vi "Create Virtual Folder (Project Item In).vi"(8 "error in":errorcluster, 10 "Item to Find":string, 11 "ProjectItem In":refnum<vi>) -> (0 "error out":errorcluster, 3 "ProjectItem out":refnum<vi>)   [LabVIEW 2014, in "SPI Engine Scripting.lvlib"]
uses:
  SPI Engine Scripting.lvlib
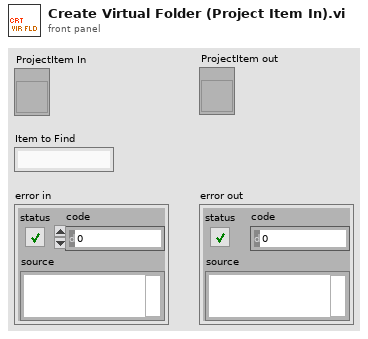
[diagram p1: front panel]
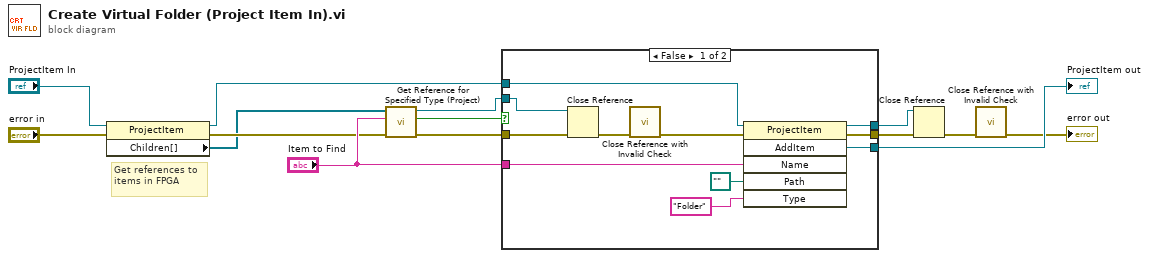
[diagram p0: block diagram]
diagram:
  # "Get references to items in FPGA"
  n1 = property class="ProjectItem"(reference="ProjectItem In", error in="error in") -> (reference out=w3:refnum<vi>, error out=w11:errorcluster, "Children[]"=w7:refnum<vi>[])
  n2 = call "Get Reference for Specified Type (Project).vi"("error in (no error)"=w11, "Type to Find"="Item to Find", "Array of References"=w7) -> ("error out"=w9:errorcluster, "Item Found"=w8:bool, "Project Item"=w10:refnum<vi>)  [unwired: 6 in]
  n3 = case shown="False" w8 {
    tunnel: [w21 w27] -> w14
    tunnel: w9 -> [w17 w28]
    tunnel: w10 -> [w15 w27]
    tunnel: [w22 w28] -> w5
    tunnel: "Item to Find" -> [w23 _]
    tunnel: [w20 w26] -> w4
    tunnel: w3 -> [w19 w26]
    frame False {
      n4 = Close Reference(reference=w15, error in (no error)=w17) -> (error out=w18:errorcluster)
      n5 = call "Close Reference with Invalid Check.vi"("error in (no error)"=w18) -> ("error out"=w16:errorcluster)  [unwired: 10 in]
      n6 = invoke class="ProjectItem" method="AddItem"(reference=w19, error in=w16, "Name"=w23, "Path"=path "", "Type"="Folder") -> (reference out=w20:refnum<vi>, error out=w22:errorcluster, "AddItem"=w21:refnum<vi>)  [unwired: 1 in, 3 out]
    }
    frame True {
    }
  }
  "ProjectItem out" <- w14
  n7 = Close Reference(reference=w4, error in (no error)=w5) -> (error out=w2:errorcluster)
  n8 = call "Close Reference with Invalid Check.vi"("error in (no error)"=w2) -> ("error out"=→"error out":errorcluster)  [unwired: 10 in]
